vi "InsertDataSampleInfo.vi"(8 "error in":errorcluster, 11 "检测电极":T1) -> (0 "error out":errorcluster)   [LabVIEW 2014, in "DataBase.lvlib"]
uses:
  DataBase.lvlib
  <vilib>/addons/database/Connection.llb/DB Tools Open Connec (String).vi
  <vilib>/addons/database/Connection.llb/Conn Execute.vi
  <vilib>/addons/database/Recordset.llb/Rec Destroy - Connection.vi
  <vilib>/addons/database/NI_Database_API.lvlib
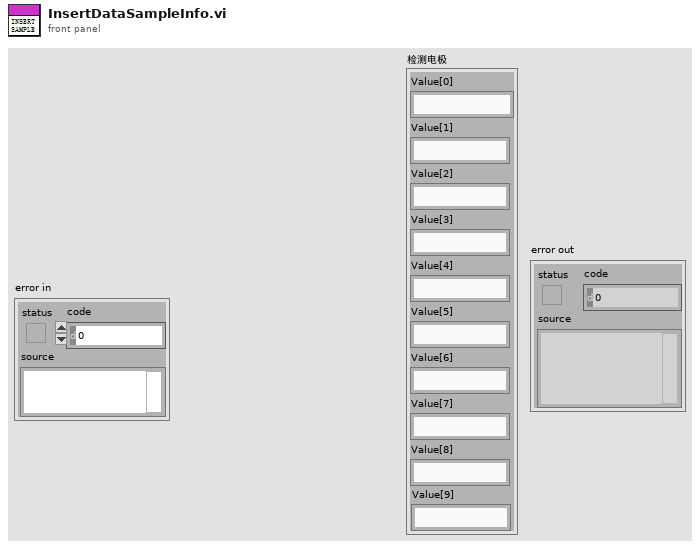
[diagram p1: front panel]
types:
  T1 = cluster{"Value[0]":string, "Value[1]":string, "Value[2]":string, "Value[3]":string, "Value[4]":string, "Value[5]":string, "Value[6]":string, "Value[7]":string, "Value[8]":string, "Value[9]":string}
  T2 = typedef "NI_Database_API.lvlib/Conn ObjectReference.ctl" = refnum<k1>
  T3 = typedef "NI_Database_API.lvlib/Rec ObjectReference.ctl" = refnum<k1>
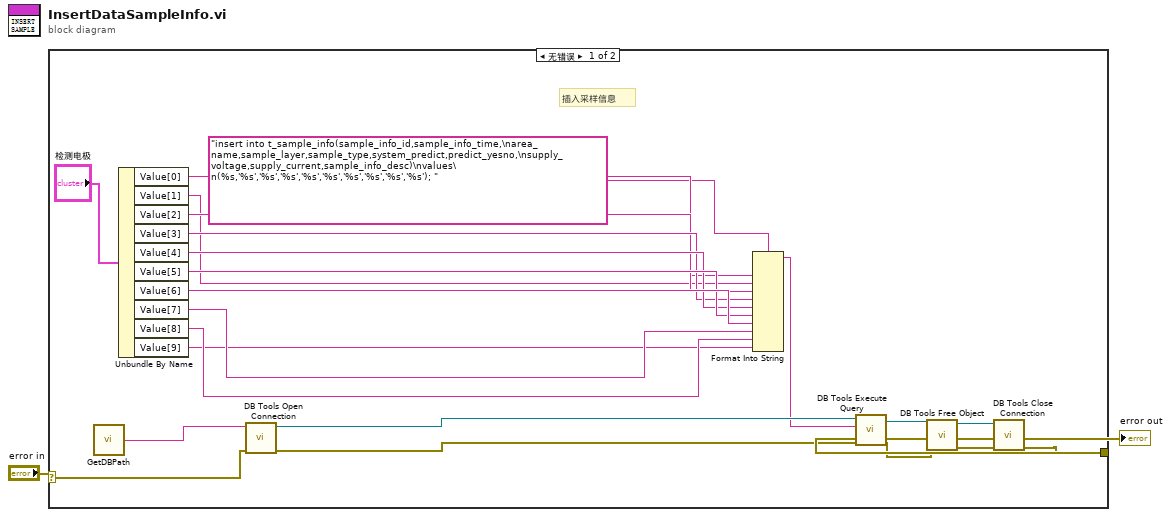
[diagram p0: block diagram]
diagram:
  n1 = case shown="无错误" "error in" {
    selector: "error in" -> [w20 w25]
    tunnel: [w3 w25] -> w1
    frame No Error {
      # "插入采样信息"
      n2 = call "GetDBPath.vi"() -> ("Connection"=w19:string)  [unwired: 1 in]
      n3 = Unbundle By Name("检测电极") -> ("Value[0]"=w8:string, "Value[1]"=w9:string, "Value[2]"=w10:string, "Value[3]"=w11:string, "Value[4]"=w12:string, "Value[5]"=w13:string, "Value[6]"=w14:string, "Value[7]"=w15:string, "Value[8]"=w16:string, "Value[9]"=w4:string)
      n4 = call-poly <vilib>:"DB Tools Open Connection.vi"("error in (no error)"=w20, "connection information"=w19) -> ("error out"=w23:errorcluster, "connection reference"=w24:T2)  [unwired: 6 in]
      n5 = Format Into String(format string="insert into t_sample_info(sample_info_id,sample_info_time,\narea_name,sample_layer,sample_type,system_predict,predict_yesno,\nsupply_voltage,supply_current,sample_info_desc)\nvalues\n(%s,'%s','%s','%s','%s','%s','%s','%s','%s','%s'); ", w8, w9, w10, w11, w12, w13, w14, w15, w16, w4) -> (resulting string=w5:string)  [unwired: 2 in, 1 out]
      n6 = call-poly <vilib>:"DB Tools Execute Query.vi"("error in (no error)"=w23, "SQL query"=w5, "connection reference"=w24) -> ("error out"=w17:errorcluster, "recordset reference"=w18:T3)  [unwired: 5 in]
      n7 = call-poly <vilib>:"DB Tools Free Object.vi"("error in (no error)"=w17, "recordset reference"=w18) -> ("error out"=w22:errorcluster, "connection reference"=w21:T2)  [unwired: 8 in]
      n8 = call <vilib>:"DB Tools Close Connection.vi"("error in (no error)"=w22, "connection reference"=w21) -> ("error out"=w3:errorcluster)  [unwired: 5 in]
    }
    frame Error {
    }
  }
  "error out" <- w1
